vi "Teleop.vi"(10 "Match Info":T1={"Autonomous Elapsed Seconds"=0.0, "TeleOp Elapsed Seconds"=0.0, "Disabled Elapsed Seconds"=0.0, "Visited Autonomous"=FALSE, "Visited TeleOp"=FALSE, "Visited Disabled"=FALSE, "Autonomous Settings"={"Autonomous Style"=enum."Independent", "VI Refnum"=refnum}}, 11 "Call Context":T2) -> ()   [LabVIEW 2015]
doc: "This VI is called for each TeleOp packet received from the DS where the robot is not disabled. It is often used to read from the joysticks and update I/O or to update setpoints for timed control loops. It should complete and return within 20 milliseconds or it may miss DS packets."
uses:
  <vilib>/Rock Robotics/WPI/DriverStation/WPI_DriverStationDerivedRobotMode.ctl
  <vilib>/Rock Robotics/WPI/DriverStation/WPI_DriverStationMatch Info.ctl
  <vilib>/Rock Robotics/WPI/Joystick/WPI_JoystickAxis.ctl
  Robot Global Data.vi
  <vilib>/Rock Robotics/WPI/Joystick/WPI_JoystickGetSetRefNum.vi
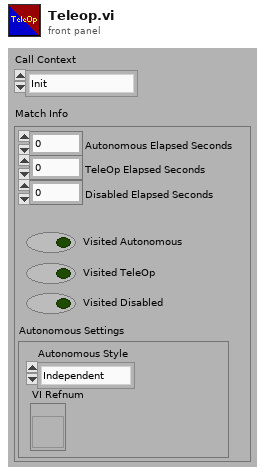
[diagram p1: front panel]
types:
  T1 = typedef "WPI_DriverStationMatch Info.ctl" = cluster{"Autonomous Elapsed Seconds":dbl, "TeleOp Elapsed Seconds":dbl, "Disabled Elapsed Seconds":dbl, "Visited Autonomous":bool, "Visited TeleOp":bool, "Visited Disabled":bool, "Autonomous Settings":cluster{"Autonomous Style":enum16{"Iterative", "Independent"}, "VI Refnum":refnum<vi>}}
  T2 = typedef "WPI_DriverStationDerivedRobotMode.ctl" = enum16{"Init", "Execute", "Stop"}
  T3 = typedef "WPI_JoystickAxis.ctl" = enum16{"Axis 1", "Axis 2", "Axis 3", "Axis 4", "Axis 5", "Axis 6"}
  T4 = typedef "WPI_JoystickDevRef.ctl" = cluster{"Device":T5}
  T5 = typedef "WPI_JoystickDeviceEnum.ctl" = enum16{"USB 0", "USB 1", "USB 2", "USB 3", "USB 4", "USB 5"}
  T6 = typedef "WPI_MotorControlDeviceRef.ctl" = cluster{"DeviceStatus":errorcluster, "Type":enum16{"PWM", "CAN"}, "PWM":cluster{"Digital Module":T7, "PWM Channel":T8, "DeadBand":T9}, "CAN":cluster{"Device Number":u8, "Control Mode":T10, "Semaphore":T11, "Max Vout":dbl}, "Invert":bool, "TransformRef":T12, "InvTransformRef":T12}
  T7 = typedef "FPGA_TypedefDigitalModule.ctl" = enum16{"Digital Module 1", "Digital Module 2"}
  T8 = typedef "FPGA_DIOPWMChannel.ctl" = enum8{"PWM 1", "PWM 2", "PWM 3", "PWM 4", "PWM 5", "PWM 6", "PWM 7", "PWM 8", "PWM 9", "PWM 10", "Invalid"}
  T9 = typedef "WPI_PWMDeadband.ctl" = cluster{"Name":string, "maxPositivePwm":i32, "minPositivePwm":i32, "centerPwm":i32, "maxNegativePwm":i32, "minNegativePwm":i32, "angularRange":u16}
  T10 = typedef "WPI_CANJaguar_ControlMode.ctl" = enum8{"Percent VBus", "Current", "Speed", "Position", "Voltage"}
  T11 = typedef "Semaphore RefNum" = refnum<k1>
  T12 = typedef "WPI_PWMTransform_ConPane.ctl" = refnum<vi>
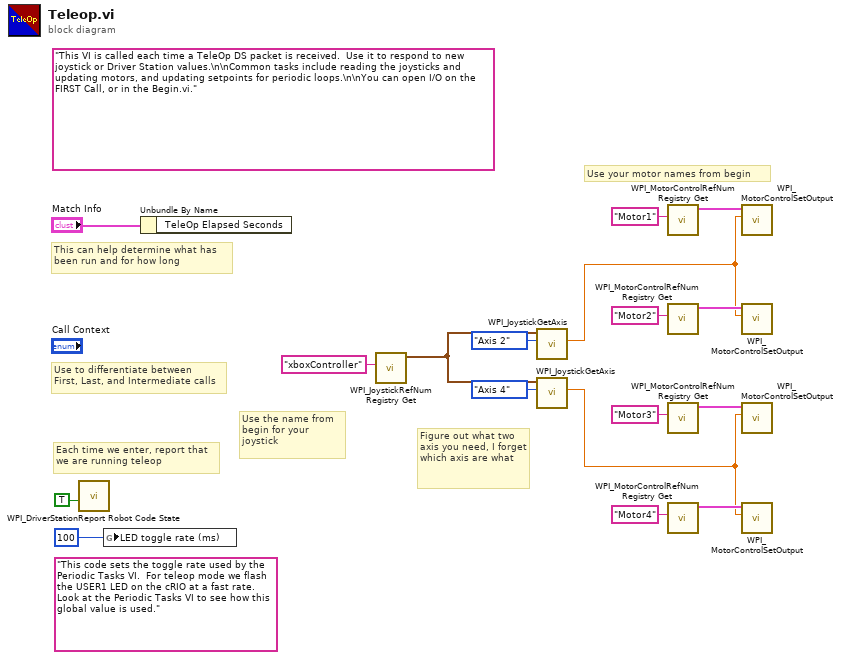
[diagram p0: block diagram]
diagram:
  (unwired) "This code sets the toggle rate used by the Periodic Tasks VI.  For teleop mode we flash the USER1 LED on the cRIO at a fast rate.  Look at the Periodic Tasks VI to see how this global value is used."
  (unwired) "This VI is called each time a TeleOp DS packet is received.  Use it to respond to new joystick or Driver Station values.\n\nCommon tasks include reading the joysticks and updating motors, and updating setpoints for periodic loops.\n\nYou can open I/O on the FIRST Call, or in the Begin.vi."
  # "Figure out what two axis you need, I forget which axis are what"
  # "Use your motor names from begin"
  # "Use the name from begin for your joystick"
  # "Each time we enter, report that\nwe are running teleop"
  # "Use to differentiate between\nFirst, Last, and Intermediate calls"
  # "This can help determine what has\nbeen run and for how long"
  n1 = call <vilib>:"WPI_DriverStationReport Robot Code State.vi"("TeleOp"=TRUE ("Autonomous")) -> ()  [unwired: 10 in, 1 out]
  n2 = global write "Robot Global Data.vi" "LED toggle rate (ms)"(u32 100 ("LED ms toggle rate")) -> ()
  n3 = Unbundle By Name("Match Info") -> ()  [unwired: 1 out]
  n4 = call <vilib>:"WPI_JoystickRefNum Registry Get.vi"("refnum name"="xboxController") -> ("JoystickDevRef"=w6:T4)  [unwired: 9 in, 1 out]
  n5 = call <vilib>:"WPI_JoystickGetAxis.vi"("Axis"=WPI_JoystickAxis."Axis 2", "JoystickDevRef"=w6) -> ("Value"=w4:dbl)  [unwired: 8 in, 1 out]
  n6 = call <vilib>:"WPI_JoystickGetAxis.vi"("Axis"=WPI_JoystickAxis."Axis 4", "JoystickDevRef"=w6) -> ("Value"=w5:dbl)  [unwired: 8 in, 1 out]
  n7 = call <vilib>:"WPI_MotorControlRefNum Registry Get.vi"("refnum name"="Motor1") -> ("MotorControlDevRef"=w13:T6)  [unwired: 9 in, 1 out]
  n8 = call <vilib>:"WPI_MotorControlRefNum Registry Get.vi"("refnum name"="Motor2") -> ("MotorControlDevRef"=w11:T6)  [unwired: 9 in, 1 out]
  n9 = call <vilib>:"WPI_MotorControlRefNum Registry Get.vi"("refnum name"="Motor3") -> ("MotorControlDevRef"=w12:T6)  [unwired: 9 in, 1 out]
  n10 = call <vilib>:"WPI_MotorControlRefNum Registry Get.vi"("refnum name"="Motor4") -> ("MotorControlDevRef"=w14:T6)  [unwired: 9 in, 1 out]
  n11 = call <vilib>:"WPI_MotorControlSetOutput.vi"("Output"=w4, "MotorControlDevRef"=w13) -> ()  [unwired: 7 in, 3 out]
  n12 = call <vilib>:"WPI_MotorControlSetOutput.vi"("Output"=w4, "MotorControlDevRef"=w11) -> ()  [unwired: 7 in, 3 out]
  n13 = call <vilib>:"WPI_MotorControlSetOutput.vi"("Output"=w5, "MotorControlDevRef"=w12) -> ()  [unwired: 7 in, 3 out]
  n14 = call <vilib>:"WPI_MotorControlSetOutput.vi"("Output"=w5, "MotorControlDevRef"=w14) -> ()  [unwired: 7 in, 3 out]
